vi "CheckWinDiag(SubVI).vi"(11 "Array":string[][](array[string])) -> (3 "x .or. y?":bool)   [LabVIEW 2020]
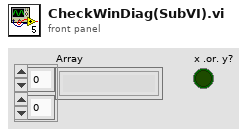
[diagram p1: front panel]
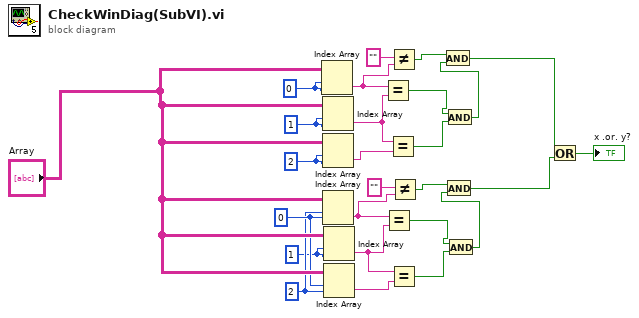
[diagram p0: block diagram]
diagram:
  w15 = 2
  w14 = 1
  w16 = 0
  w3 = 2
  w2 = 1
  w1 = 0
  n1 = Index Array(array="Array", index (row)=w1, index (col)=w1) -> (element=w9:string)
  n2 = Index Array(array="Array", index (row)=w2, index (col)=w2) -> (element=w4:string)
  n3 = Index Array(array="Array", index (row)=w3, index (col)=w3) -> (element=w23:string)
  n4 = Index Array(array="Array", index (row)=w15, index (col)=w16) -> (element=w22:string)
  n5 = Index Array(array="Array", index (row)=w14, index (col)=w14) -> (element=w20:string)
  n6 = Index Array(array="Array", index (row)=w16, index (col)=w15) -> (element=w21:string)
  n7 = Equal?(x=w9, y=w4) -> (x = y?=w5:bool)
  n8 = Equal?(x=w22, y=w20) -> (x = y?=w13:bool)
  n9 = Equal?(x=w4, y=w23) -> (x = y?=w6:bool)
  n10 = Not Equal?(x="", y=w9) -> (x != y?=w7:bool)
  n11 = Equal?(x=w20, y=w21) -> (x = y?=w12:bool)
  n12 = Not Equal?(x="", y=w22) -> (x != y?=w11:bool)
  n13 = And(x=w5, y=w6) -> (x .and. y?=w17:bool)
  n14 = And(x=w7, y=w17) -> (x .and. y?=w24:bool)
  n15 = And(x=w13, y=w12) -> (x .and. y?=w18:bool)
  n16 = And(x=w11, y=w18) -> (x .and. y?=w25:bool)
  n17 = Or(x=w24, y=w25) -> (x .or. y?=→"x .or. y?":bool)
